vi "ITestSettings Raw Configuration to Specific Data Type.vi"(8 "error in (no error)":errorcluster, 10 "Raw Config Data":refnum<class "String Database.lvclass">[](array[class]), 11 "2SG_IMD Test Settings in":refnum<class "2SG_IMD Test Settings.lvclass">) -> (0 "error out":errorcluster, 3 "2SG_IMD Test Settings out":refnum<class "2SG_IMD Test Settings.lvclass">)   [LabVIEW 2016, in "2SG_IMD Test Settings.lvlib" / "2SG_IMD Test Settings.lvclass"]
uses:
  2SG_IMD Test Settings.lvclass
  C:/Projects/STS/Common/Sequence Automation/Plugins/Test Settings/ITestSettings.lvlibp/ITestSettings.lvclass
  Plugins/String Database.lvlibp/String Database.lvclass
  Controls/2SG_IMD Settings Cluster.ctl
  Plugins/Test Settings/ITestSettings.lvlibp/Protected Methods/Read Configuration Dictionary.vi
  Plugins/Test Settings/ITestSettings.lvlibp/Protected Methods/Write Configuration Dictionary.vi
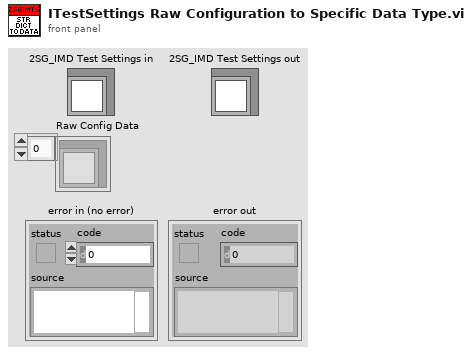
[diagram p1: front panel]
types:
  T1 = typedef "2SG_IMD Test Settings.lvlib/2SG_IMD Test Settings.lvclass/2SG_IMD Settings Cluster.ctl" = cluster{"SG Frequency Offset":dbl, "SA Frequency Offset":dbl, "SA Reference Level":dbl, "2SG Frequency":dbl, "2SG Relative Power Level":dbl, "2SG Waveform Name":string}
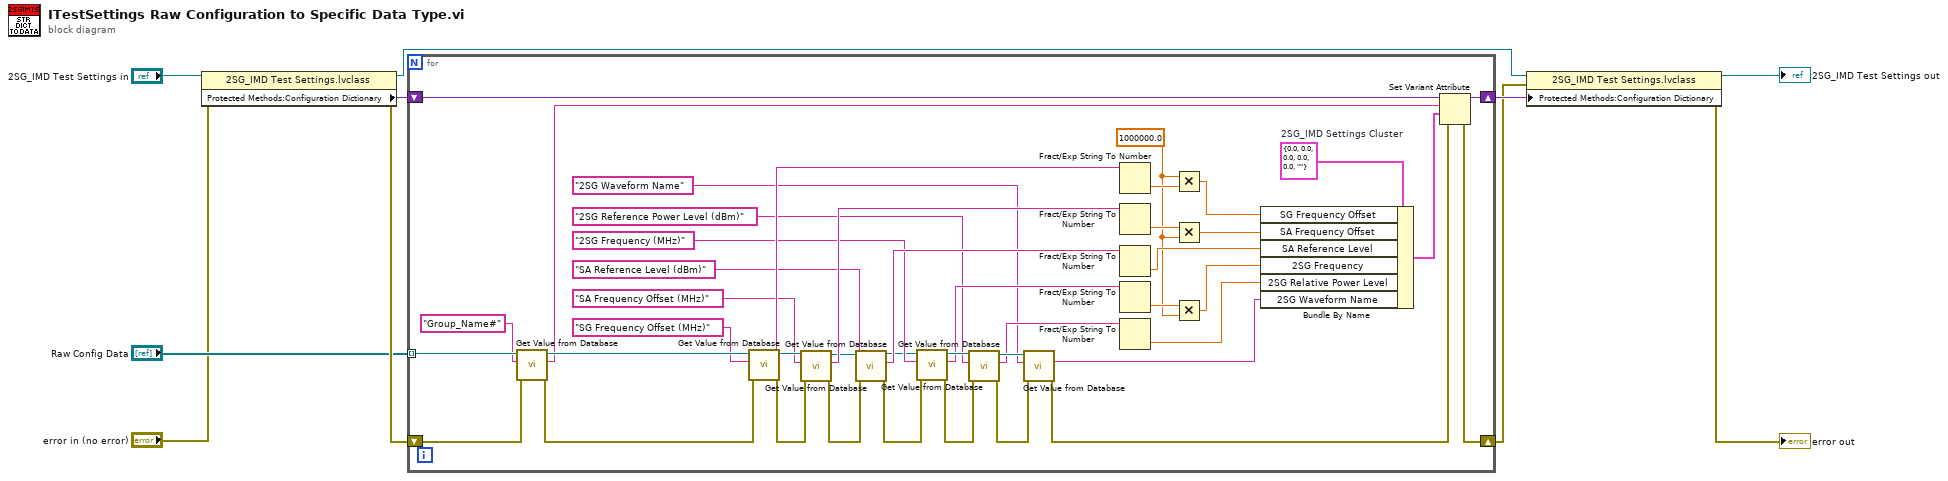
[diagram p0: block diagram]
diagram:
  n1 = property class="2SG_IMD Test Settings.lvclass"(reference="2SG_IMD Test Settings in", error in="error in (no error)") -> (reference out=w7:refnum<class "2SG_IMD Test Settings.lvclass">, error out=w9:errorcluster, "Protected Methods:Configuration Dictionary"=w10:variant)
  n2 = for {
    shift-right: [w52] -> w6
    shift-left: w9 -> [w49]
    shift-right: [w51] -> w8
    shift-left: w10 -> [w53]
    tunnel: "Raw Config Data" -> [w50] mode=indexing
    w28 = T1 {"SG Frequency Offset"=0.0, "SA Frequency Offset"=0.0, "SA Reference Level"=0.0, "2SG Frequency"=0.0, "2SG Relative Power Level"=0.0, "2SG Waveform Name"=""}  # 2SG_IMD Settings Cluster
    w18 = 1000000.0 ("x")
    n3 = call "Get Value from Database.vi"("error in (no error)"=w49, "Entry Name"="Group_Name#", "Message in"=w50) -> ("error out"=w46:errorcluster, "Entry Value"=w43:string, "Message out"=w47:refnum<class "String Database.lvclass">)  [unwired: 5 in, 1 out]
    n4 = call "Get Value from Database.vi"("error in (no error)"=w46, "Entry Name"="SG Frequency Offset (MHz)", "Message in"=w47) -> ("error out"=w44:errorcluster, "Entry Value"=w40:string, "Message out"=w45:refnum<class "String Database.lvclass">)  [unwired: 5 in, 1 out]
    n5 = call "Get Value from Database.vi"("error in (no error)"=w44, "Entry Name"="SA Frequency Offset (MHz)", "Message in"=w45) -> ("error out"=w32:errorcluster, "Entry Value"=w34:string, "Message out"=w33:refnum<class "String Database.lvclass">)  [unwired: 5 in, 1 out]
    n6 = call "Get Value from Database.vi"("error in (no error)"=w32, "Entry Name"="SA Reference Level (dBm)", "Message in"=w33) -> ("error out"=w22:errorcluster, "Entry Value"=w30:string, "Message out"=w20:refnum<class "String Database.lvclass">)  [unwired: 5 in, 1 out]
    n7 = call "Get Value from Database.vi"("error in (no error)"=w22, "Entry Name"="2SG Frequency (MHz)", "Message in"=w20) -> ("error out"=w25:errorcluster, "Entry Value"=w16:string, "Message out"=w26:refnum<class "String Database.lvclass">)  [unwired: 5 in, 1 out]
    n8 = call "Get Value from Database.vi"("error in (no error)"=w25, "Entry Name"="2SG Reference Power Level (dBm)", "Message in"=w26) -> ("error out"=w24:errorcluster, "Entry Value"=w14:string, "Message out"=w27:refnum<class "String Database.lvclass">)  [unwired: 5 in, 1 out]
    n9 = call "Get Value from Database.vi"("error in (no error)"=w24, "Entry Name"="2SG Waveform Name", "Message in"=w27) -> ("error out"=w23:errorcluster, "Entry Value"=w11:string)  [unwired: 5 in, 2 out]
    n10 = Fract/Exp String To Number(string=w40) -> (number=w39:dbl)  [unwired: 3 in, 1 out]
    n11 = Fract/Exp String To Number(string=w34) -> (number=w36:dbl)  [unwired: 3 in, 1 out]
    n12 = Fract/Exp String To Number(string=w30) -> (number=w29:dbl)  [unwired: 3 in, 1 out]
    n13 = Fract/Exp String To Number(string=w16) -> (number=w19:dbl)  [unwired: 3 in, 1 out]
    n14 = Fract/Exp String To Number(string=w14) -> (number=w13:dbl)  [unwired: 3 in, 1 out]
    n15 = Multiply(x=w18, y=w39) -> (x*y=w38:dbl)
    n16 = Multiply(x=w36, y=w18) -> (x*y=w35:dbl)
    n17 = Multiply(x=w19, y=w18) -> (x*y=w17:dbl)
    n18 = Bundle By Name(cluster=w28, "SG Frequency Offset"=w38, "SA Frequency Offset"=w35, "SA Reference Level"=w29, "2SG Frequency"=w17, "2SG Relative Power Level"=w13, "2SG Waveform Name"=w11) -> (w42:T1)
    n19 = Set Variant Attribute(Variant=w53, name=w43, value=w42, error in=w23) -> (Variant out=w51:variant, error out=w52:errorcluster)  [unwired: 1 out]
  }
  n20 = property class="2SG_IMD Test Settings.lvclass"(reference=w7, error in=w6, "Protected Methods:Configuration Dictionary"=w8) -> (reference out=→"2SG_IMD Test Settings out":refnum<class "2SG_IMD Test Settings.lvclass">, error out=→"error out":errorcluster)
